vi "Main_spb_framegr.vi"() -> ()   [LabVIEW 2018]
uses:
  <vilib>/Platform/TimedLoop/XDataNode/timing_clust.ctl
  <vilib>/Platform/TimedLoop/XDataNode/nitl_modes.ctl
  <vilib>/Platform/TimedLoop/XDataNode/wakeup.ctl
  <vilib>/rvi/eio/common/nirviEmuTemplateMethod_errors.vi
  <vilib>/rvi/Emulation/niFpgaGetClockAttributes.vi
  <vilib>/rvi/Emulation/niFpgaSctlEmulationGetInTimedLoop.vi
  <vilib>/rvi/Emulation/niFpgaEmulationReportErrorSimple.vi
  <vilib>/rvi/Emulation/niFpgaProcessEmulError.vi
  <vilib>/rvi/Emulation/niFpgaCriticalErrorInLSC.vi
  <vilib>/eio/EIONode/EIONode.xnode
  <vilib>/Platform/TimedLoop/XDataNode/XDataNode.xnode
  <vilib>/Platform/TimedLoop/XDataNode/XDNodeRunTimeDep.lvlib
panel:
  in  "Фильм":bool
  in  "6":i8=6
  in  "12":i8=12
  in  "3":i8=3
  in  "RELAY_18_IN1":bool
  in  "RELAY_18_IN2":bool
  in  "RELAY_28_IN1":bool
  in  "RELAY_28_IN2":bool
  in  "RELAY_30_IN1":bool
  in  "RELAY_30_IN2":bool
  out "I":i32
  in  "Свет до":u32
  in  "Свет от":u32
  in  "Задержка":u32
  in  "Линейки":bool
  in  "Свет":bool
  in  "Строка триггер":u16=1200
  in  "Остановка основного цикла":bool
  in  "Горизонталы":i32=1048
  in  "H1_1":i8=10
  in  "H1_2":i8=36
  in  "H2_1":i8=3
  in  "H2_2":i8=28
  in  "H3_1":i8=20
  in  "H3_2":i8=45
  in  "RG_1":i8=6
  in  "RG_2":i8=16
  in  "48":i8=48
  in  "После H, мкс":u16=15
  in  "CDS1_1":i8=20
  in  "CDS1_2":i8=24
  in  "CDS2_1":i8=36
  in  "CDS2_2":i8=47
  in  "ADC_1":i8=20
  in  "ADC_2":i8=41
  in  "Задержка после переноса строки, мкс":u16=15
  in  "1800":i16=1800
  in  "S3_1":i16=50
  in  "S3_2":i16=950
  in  "S2_1":i16=600
  in  "S2_2":i16=1500
  in  "S1_1":i16=300
  in  "S1_2":i16=1200
  in  "Сколько строк?":i32=2047
  in  "Read(T)/Write(F)":bool
  in  "Enum":T1(ring)
  in  "Write Data":bool[](array[boolean])=[FALSE, FALSE, FALSE, FALSE, FALSE, FALSE, FALSE, FALSE, FALSE]
  in  "8":i8=8
  out "READ":bool[](array[boolean])
  in  "18":i8=18
  in  "7":i8=7
  in  "18_1":i8=18
  in  "Конфигурация":bool
  in  "Кадр":bool
  in  "Command array":bool[](array[boolean])=[FALSE, FALSE, FALSE, FALSE, FALSE, FALSE, FALSE, FALSE, FALSE, FALSE, FALSE, FALSE, FALSE, FALSE, FALSE, FALSE, FALSE]
  # "Чтобы записать кадр в память,\nсначала \"Кадр в память\", затем\nкнопка \"Автомат\""
  # "8"
  # "0"
  # "8"
  # "0"
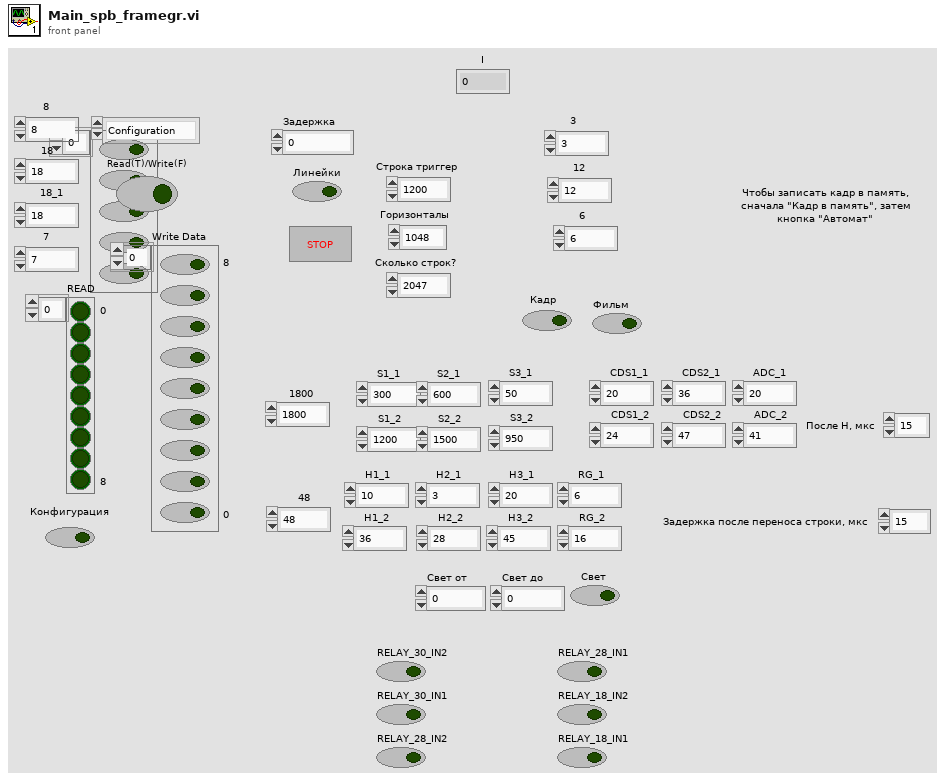
[diagram p1: front panel]
types:
  T1 = enum16{"Configuration", "MUX", "RED PGA", "GREEN PGA", "BLUE PGA", "RED OFF", "GREEN OFF", "BLUE OFF"}
  T2 = typedef "XDNodeRunTimeDep.lvlib/timing_clust.ctl" = cluster{"Expected End [f-1]":u64, "Actual End [f-1]":u64, "Finished Late? [f-1]":bool, "Expected End [i-1]":u64, "Actual End [i-1]":u64, "Finished Late? [i-1]":bool, "Expected Start [i]":u64, "Actual Start [i]":u64, "Expected Start [f]":u64, "Actual Start [f]":u64, "Source Name":string, "Structure Name":string, "Period":i64, "Deadline":i64, "Offset":i64, "Start":i64, "Priority":i32, "Timeout":i32, "Mode":T3, "Wakeup Reason":T4, "Error":errorcluster, "Source Type":string, "Secondary Source Type":string, "Global End Time":u64, "Global Start Time":u64, "Frame Duration":u64, "Iteration Duration":u64, "Assigned CPU":i32, "I/O Scan Engine Mode":u32}
  T3 = typedef "XDNodeRunTimeDep.lvlib/nitl_modes.ctl" = enum32{"No Change", "Process missed periods, maintain original phase", "Discard missed periods, maintain original phase", "Process missed periods, ignore original phase", "Discard missed periods, ignore original phase"}
  T4 = typedef "XDNodeRunTimeDep.lvlib/wakeup.ctl" = enum32{"Normal", "Aborted", "Asynchronous wakeup", "Timing source error", "Timed loop error", "Timeout"}
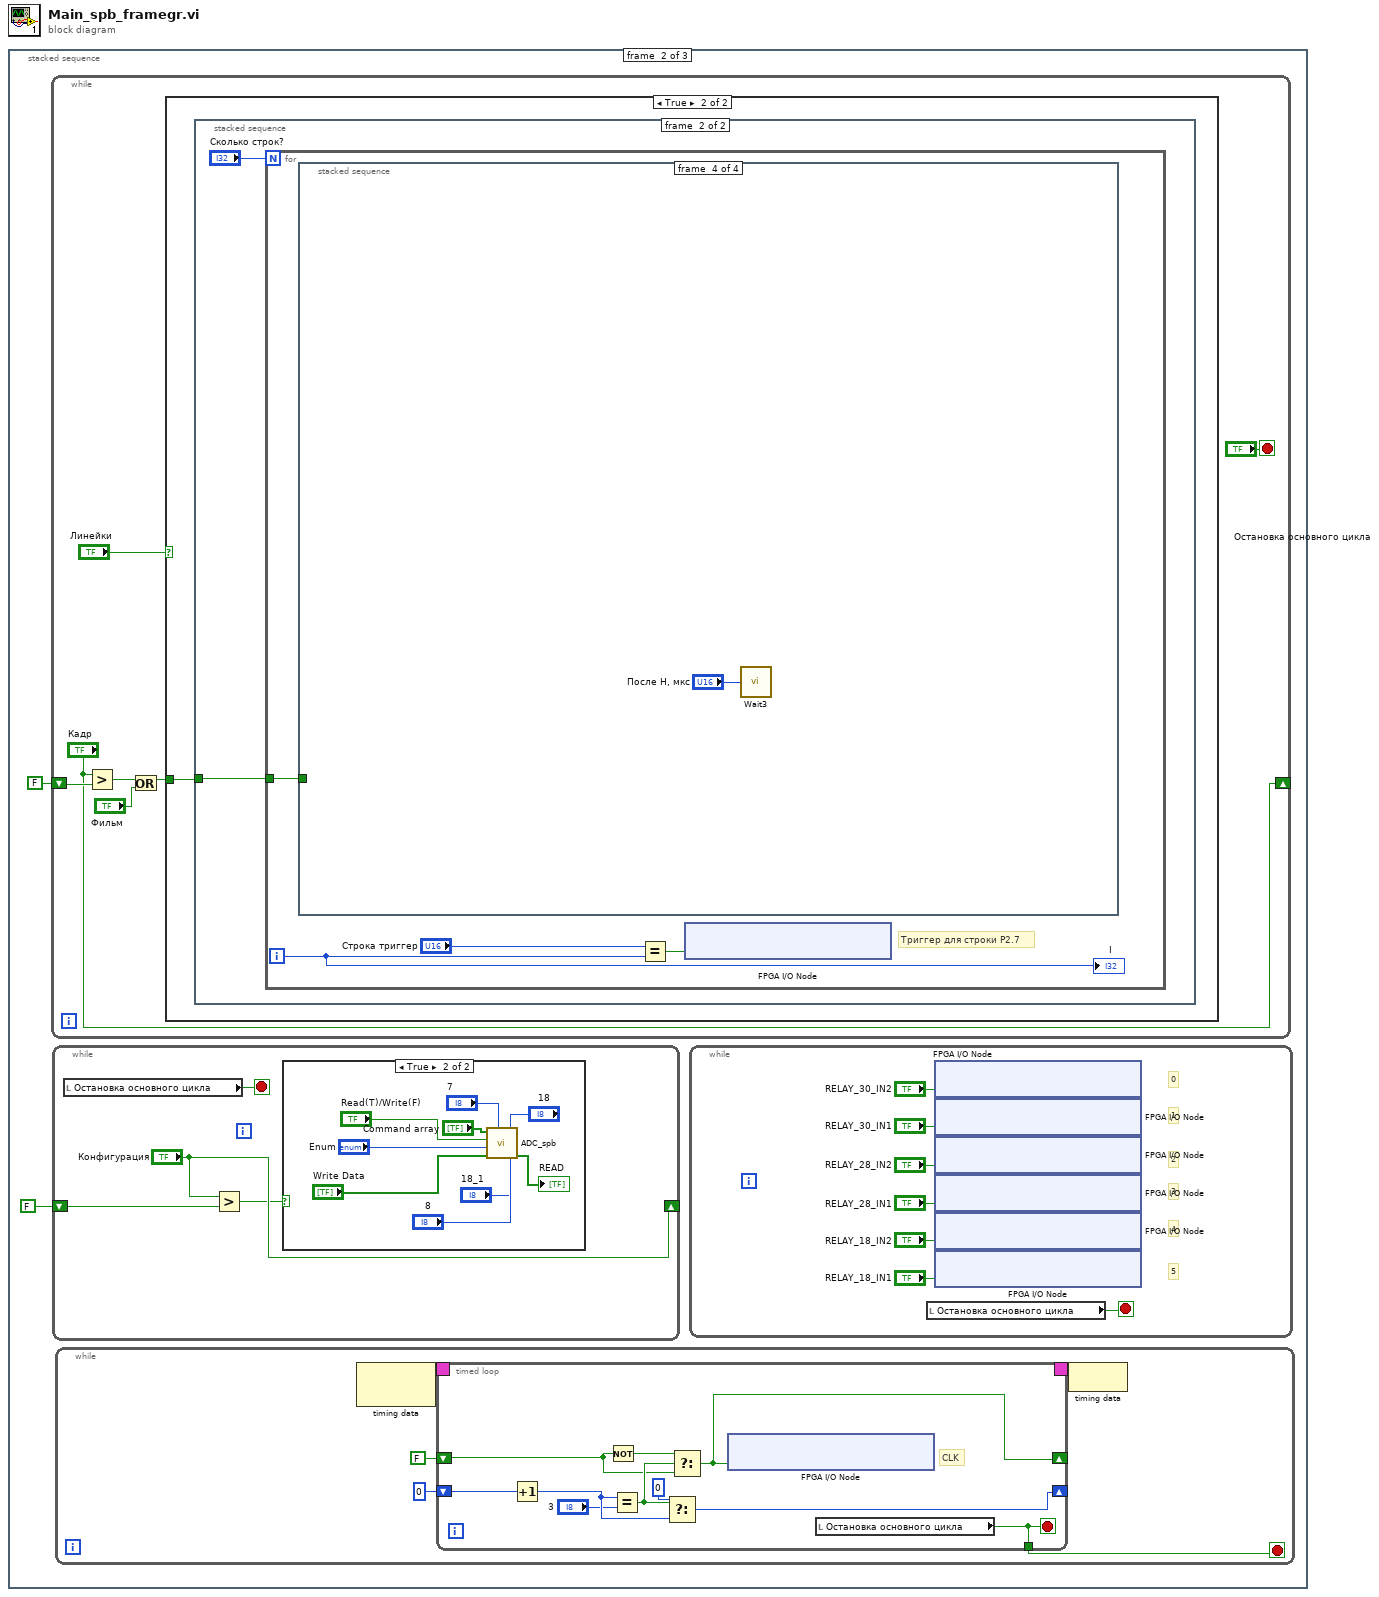
[diagram p0: block diagram]
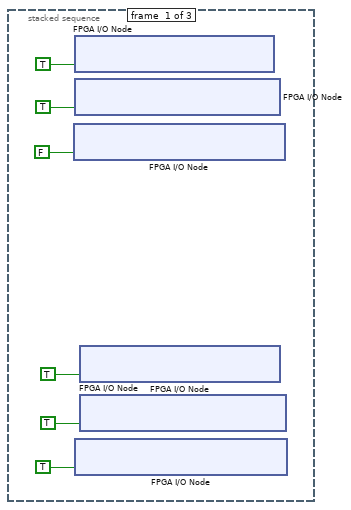
[diagram p2: hidden frame]
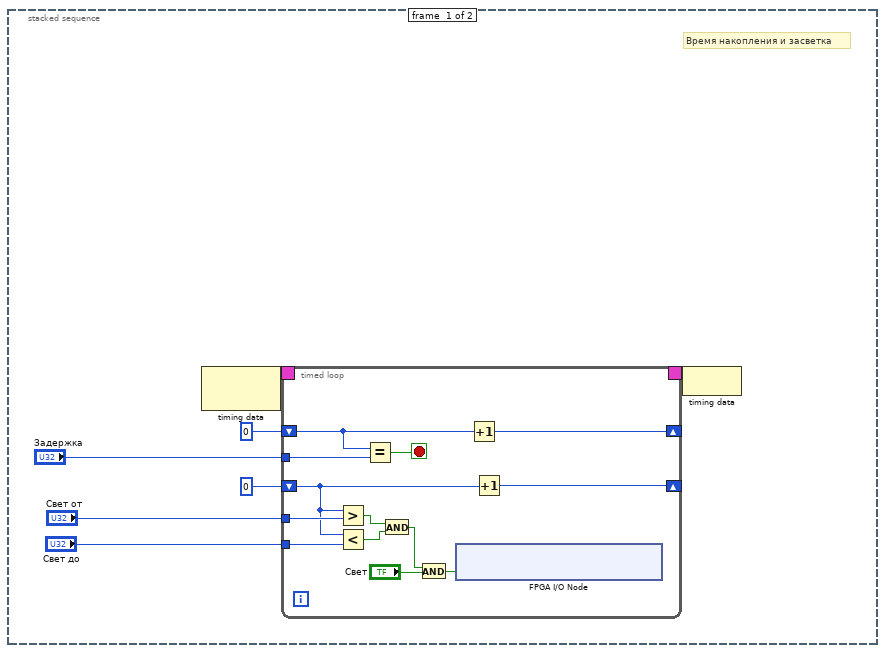
[diagram p4: hidden frame]
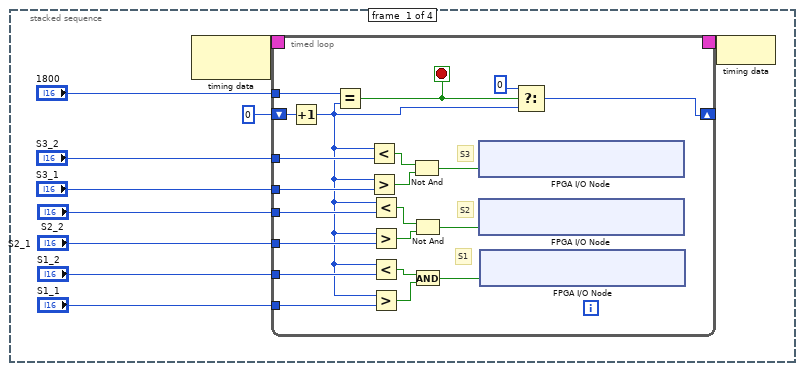
[diagram p5: hidden frame]
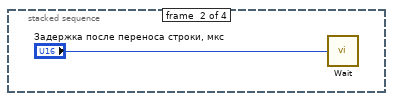
[diagram p6: hidden frame]
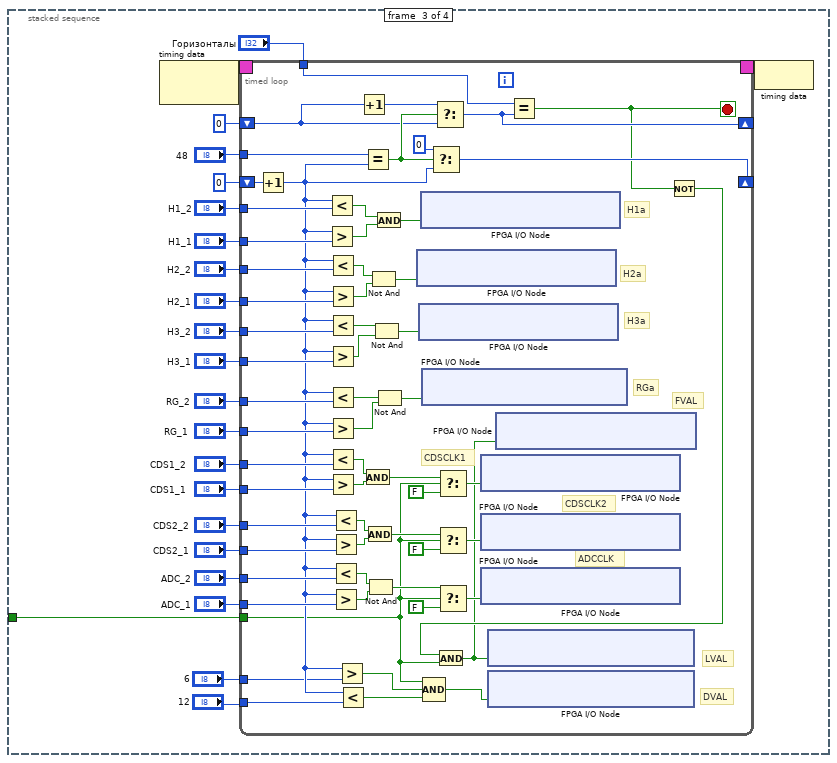
[diagram p7: hidden frame]
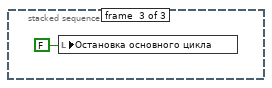
[diagram p9: hidden frame]
diagram:
  n1 = stacked-sequence {
    frame #0 {
      n2 = xnode "FPGA I/O Node"("IO Module\\DDCB_DIO16-23_WE"=FALSE ("IO Module\\DDCB_DIO16-23_WE")) -> ()  [unwired: 1 in, 1 out]
      n3 = xnode "FPGA I/O Node"("IO Module\\DDCB_DIO0-7_WE"=TRUE) -> ()  [unwired: 1 in, 1 out]
      n4 = xnode "FPGA I/O Node"("IO Module\\DDCB_DIO8-15_WE"=TRUE) -> ()  [unwired: 1 in, 1 out]
      n5 = xnode "FPGA I/O Node"("IO Module\\DDCA_DIO16-23_WE"=TRUE) -> ()  [unwired: 1 in, 1 out]
      n6 = xnode "FPGA I/O Node"("IO Module\\DDCA_DIO0-7_WE"=TRUE) -> ()  [unwired: 1 in, 1 out]
      n7 = xnode "FPGA I/O Node"("IO Module\\DDCA_DIO8-15_WE"=TRUE) -> ()  [unwired: 1 in, 1 out]
    }
    frame #1 {
      n8 = while {
        shift-right: ["Кадр"] -> _
        shift-left: FALSE ("Кадр в память") -> [w39]
        stop <- "Остановка основного цикла" stop-if-true
        n9 = Greater?(x="Кадр", y=w39) -> (0:w37:bool)
        n10 = Or(x=w37, y="Фильм") -> (x .or. y?=w36:bool)
        n11 = case shown="True" "Линейки" {
          tunnel: w36 -> [_ w42]
          frame False {
          }
          frame True {
            n12 = stacked-sequence {
              tunnel: w42 -> [_ w68]
              frame #0 {
                # "Время накопления и засветка"
                n13 = node-c288() -> (w49:T2)  [unwired: 1 in]
                n14 = timed-loop {
                  timing: w49 -> [_]
                  timing-out: [_] -> w48
                  shift-right: [w59] -> _
                  shift-left: u32 0 -> [w60]
                  tunnel: "Задержка" -> [w62]
                  shift-right: [w53] -> _
                  shift-left: u32 0 -> [w54]
                  tunnel: "Свет от" -> [w58]
                  tunnel: "Свет до" -> [w57]
                  stop <- w61 stop-if-true
                  n15 = Greater?(x=w54, y=w58) -> (0:w56:bool)
                  n16 = Less?(x=w54, y=w57) -> (x < y?=w55:bool)
                  n17 = Equal?(x=w60, y=w62) -> (x = y?=w61:bool)
                  n18 = And(x=w56, y=w55) -> (x .and. y?=w51:bool)
                  n19 = And(x=w51, y="Свет") -> (x .and. y?=w52:bool)
                  n20 = xnode "FPGA I/O Node"("IO Module\\DDCA_DIO22_Write"=w52) -> ()  [unwired: 1 in, 1 out]
                  n21 = Increment(x=w60) -> (x+1=w59:u32)
                  n22 = Increment(x=w54) -> (x+1=w53:u32)
                }
                n23 = node-c288(w48) -> ()
              }
              frame #1 {
                n24 = for {
                  N: "Сколько строк?" -> [_]
                  tunnel: w68 -> [w70]
                  i -> [w69]
                  # "Триггер для строки Р2.7"
                  n25 = stacked-sequence {
                    tunnel: w70 -> [_ _ w111 _]
                    frame #0 {
                      n26 = node-c288() -> (w82:T2)  [unwired: 1 in]
                      n27 = timed-loop {
                        shift-right: [w101] -> _
                        shift-left: i16 0 -> [w103]
                        timing: w82 -> [_]
                        timing-out: [_] -> w81
                        tunnel: "1800" -> [w100]
                        tunnel: "S3_2" -> [w90]
                        tunnel: "S3_1" -> [w89]
                        tunnel: "S2_2" -> [w88]
                        tunnel: "S2_1" -> [w87]
                        tunnel: "S1_2" -> [w86]
                        tunnel: "S1_1" -> [w85]
                        stop <- w84 stop-if-true
                        # "S1"
                        # "S2"
                        # "S3"
                        n28 = Increment(x=w103) -> (x+1=w83:i16)
                        n29 = Equal?(x=w100, y=w83) -> (x = y?=w84:bool)
                        n30 = Less?(x=w83, y=w90) -> (x < y?=w94:bool)
                        n31 = Greater?(x=w83, y=w89) -> (0:w95:bool)
                        n32 = Less?(x=w83, y=w88) -> (x < y?=w96:bool)
                        n33 = Greater?(x=w83, y=w87) -> (0:w97:bool)
                        n34 = Less?(x=w83, y=w86) -> (x < y?=w98:bool)
                        n35 = Greater?(x=w83, y=w85) -> (0:w99:bool)
                        n36 = Not And(1:w95, 2:w94) -> (0:w93:bool)
                        n37 = Not And(1:w97, 2:w96) -> (0:w92:bool)
                        n38 = And(x=w98, y=w99) -> (x .and. y?=w91:bool)
                        n39 = xnode "FPGA I/O Node"("IO Module\\DDCB_DIO11_Write"=w93) -> ()  [unwired: 1 in, 1 out]
                        n40 = xnode "FPGA I/O Node"("IO Module\\DDCB_DIO12_Write"=w92) -> ()  [unwired: 1 in, 1 out]
                        n41 = xnode "FPGA I/O Node"("IO Module\\DDCB_DIO13_Write"=w91) -> ()  [unwired: 1 in, 1 out]
                        n42 = Select(t=i16 0, s=w84, f=w83) -> (s? t:f=w101:i16)
                      }
                      n43 = node-c288(w81) -> ()
                    }
                    frame #1 {
                      n44 = call "Wait"("Count(uSec)"="Задержка после переноса строки, мкс") -> ()  [unwired: 1 out]
                    }
                    frame #2 {
                      n45 = node-c288() -> (w131:T2)  [unwired: 1 in]
                      n46 = timed-loop {
                        timing: w131 -> [_]
                        timing-out: [_] -> w130
                        tunnel: "H1_2" -> [w187]
                        tunnel: "H1_1" -> [w186]
                        tunnel: "H2_2" -> [w191]
                        tunnel: "H2_1" -> [w190]
                        tunnel: "H3_2" -> [w189]
                        tunnel: "H3_1" -> [w188]
                        shift-right: [w180] -> _
                        shift-left: i8 0 -> [w185]
                        tunnel: "RG_2" -> [w184]
                        tunnel: "RG_1" -> [w183]
                        tunnel: "48" -> [w182]
                        tunnel: "Горизонталы" -> [w164]
                        shift-right: [w163] -> _
                        shift-left: 0 -> [w165]
                        tunnel: "CDS1_2" -> [w156]
                        tunnel: "CDS1_1" -> [w155]
                        tunnel: "CDS2_2" -> [w154]
                        tunnel: "CDS2_1" -> [w153]
                        tunnel: "ADC_2" -> [w152]
                        tunnel: "ADC_1" -> [w151]
                        tunnel: w111 -> [w135]
                        tunnel: "6" -> [w138]
                        tunnel: "12" -> [w137]
                        stop <- w134 stop-if-true
                        # "FVAL"
                        # "LVAL"
                        # "DVAL"
                        # "ADCCLK"
                        # "CDSCLK2"
                        # "CDSCLK1"
                        # "H3a"
                        # "H2a"
                        # "H1a"
                        # "RGa"
                        n47 = Increment(x=w185) -> (x+1=w139:i8)
                        n48 = Less?(x=w139, y=w187) -> (x < y?=w179:bool)
                        n49 = Greater?(x=w139, y=w186) -> (0:w178:bool)
                        n50 = Less?(x=w139, y=w191) -> (x < y?=w177:bool)
                        n51 = Greater?(x=w139, y=w190) -> (0:w176:bool)
                        n52 = Less?(x=w139, y=w189) -> (x < y?=w175:bool)
                        n53 = Greater?(x=w139, y=w188) -> (0:w174:bool)
                        n54 = Less?(x=w139, y=w184) -> (x < y?=w173:bool)
                        n55 = Greater?(x=w139, y=w183) -> (0:w172:bool)
                        n56 = Less?(x=w139, y=w156) -> (x < y?=w157:bool)
                        n57 = Greater?(x=w139, y=w155) -> (0:w158:bool)
                        n58 = Less?(x=w139, y=w154) -> (x < y?=w160:bool)
                        n59 = Greater?(x=w139, y=w153) -> (0:w159:bool)
                        n60 = Less?(x=w139, y=w152) -> (x < y?=w161:bool)
                        n61 = Greater?(x=w139, y=w151) -> (0:w162:bool)
                        n62 = Greater?(x=w139, y=w138) -> (0:w141:bool)
                        n63 = Less?(x=w139, y=w137) -> (x < y?=w140:bool)
                        n64 = Increment(x=w165) -> (x+1=w166:i32)
                        n65 = Equal?(x=w182, y=w139) -> (x = y?=w167:bool)
                        n66 = And(x=w157, y=w158) -> (x .and. y?=w148:bool)
                        n67 = And(x=w160, y=w159) -> (x .and. y?=w147:bool)
                        n68 = Not And(1:w162, 2:w161) -> (0:w146:bool)
                        n69 = Not And(1:w176, 2:w177) -> (0:w169:bool)
                        n70 = Not And(1:w174, 2:w175) -> (0:w168:bool)
                        n71 = And(x=w179, y=w178) -> (x .and. y?=w170:bool)
                        n72 = Not And(1:w172, 2:w173) -> (0:w171:bool)
                        n73 = xnode "FPGA I/O Node"("IO Module\\DDCB_DIO5_Write"=w169) -> ()  [unwired: 1 in, 1 out]
                        n74 = xnode "FPGA I/O Node"("IO Module\\DDCB_DIO6_Write"=w168) -> ()  [unwired: 1 in, 1 out]
                        n75 = xnode "FPGA I/O Node"("IO Module\\DDCB_DIO4_Write"=w170) -> ()  [unwired: 1 in, 1 out]
                        n76 = xnode "FPGA I/O Node"("IO Module\\DDCB_DIO10_Write"=w171) -> ()  [unwired: 1 in, 1 out]
                        n77 = Compound Arithmetic op=AND(w135, w141, w140) -> (w136:bool)
                        n78 = Select(t=i8 0, s=w167, f=w139) -> (s? t:f=w180:i8)
                        n79 = Select(t=w166, s=w167, f=w165) -> (s? t:f=w163:i32)
                        n80 = Select(t=w148, s=w135, f=FALSE) -> (s? t:f=w150:bool)
                        n81 = Select(t=w147, s=w135, f=FALSE) -> (s? t:f=w149:bool)
                        n82 = Select(t=w146, s=w135, f=FALSE) -> (s? t:f=w142:bool)
                        n83 = xnode "FPGA I/O Node"("IO Module\\DDCB_DIO0_Write"=w150) -> ()  [unwired: 1 in, 1 out]
                        n84 = xnode "FPGA I/O Node"("IO Module\\DDCB_DIO3_Write"=w149) -> ()  [unwired: 1 in, 1 out]
                        n85 = xnode "FPGA I/O Node"("IO Module\\DDCB_DIO1_Write"=w142) -> ()  [unwired: 1 in, 1 out]
                        n86 = xnode "FPGA I/O Node"("IO Module\\DDCA_DIO10_Write"=w136) -> ()  [unwired: 1 in, 1 out]
                        n87 = Equal?(x=w164, y=w163) -> (x = y?=w134:bool)
                        n88 = Not(x=w134) -> (.not. x?=w133:bool)
                        n89 = And(x=w133, y=w135) -> (x .and. y?=w132:bool)
                        n90 = xnode "FPGA I/O Node"("IO Module\\DDCA_DIO12_Write"=w132) -> ()  [unwired: 1 in, 1 out]
                        n91 = xnode "FPGA I/O Node"("IO Module\\DDCA_DIO8_Write"=w132) -> ()  [unwired: 1 in, 1 out]
                      }
                      n92 = node-c288(w130) -> ()
                    }
                    frame #3 {
                      n93 = call "Wait3"("Count(uSec)"="После H, мкс") -> ()  [unwired: 1 out]
                    }
                  }
                  n94 = Equal?(x="Строка триггер", y=w69) -> (x = y?=w71:bool)
                  n95 = xnode "FPGA I/O Node"("IO Module\\DDCA_DIO23_Write"=w71) -> ()  [unwired: 1 in, 1 out]
                  "I" <- w69
                }
              }
            }
          }
        }
      }
      n96 = while {
        shift-right: ["Конфигурация"] -> _
        shift-left: FALSE ("Конфигурация") -> [w199]
        stop <- w200 stop-if-true
        n97 = local read "Остановка основного цикла"() -> (w200:bool)
        n98 = Greater?(x="Конфигурация", y=w199) -> (0:w197:bool)
        n99 = case shown="True" w197 {
          frame False {
          }
          frame True {
            n100 = call "ADC_spb.vi"(1:"18_1"="18", 2:"18_1"="18_1", "8"="8", "7"="7", "Write Data"="Write Data", "Enum"="Enum", "Read(T)/Write(F)"="Read(T)/Write(F)", "Command array"="Command array") -> ("READ"=→"READ":bool[])
          }
        }
      }
      n101 = while {
        stop <- w9 stop-if-true
        n102 = node-c288() -> (w13:T2)  [unwired: 1 in]
        n103 = timed-loop {
          timing: w13 -> [_]
          timing-out: [_] -> w12
          shift-right: [w17] -> _
          shift-left: FALSE -> [w18]
          shift-right: [w15] -> _
          shift-left: i8 0 -> [w16]
          tunnel: [w14] -> w9
          stop <- w14 stop-if-true
          # "CLK"
          n104 = Increment(x=w16) -> (x+1=w22:i8)
          n105 = Not(x=w18) -> (.not. x?=w19:bool)
          n106 = Equal?(x=w22, y="3") -> (x = y?=w20:bool)
          n107 = Select(t=i8 0, s=w20, f=w22) -> (s? t:f=w15:i8)
          n108 = Select(t=w19, s=w20, f=w18) -> (s? t:f=w17:bool)
          n109 = xnode "FPGA I/O Node"("IO Module\\DDCA_DIO14_Write"=w17) -> ()  [unwired: 1 in, 1 out]
          n110 = local read "Остановка основного цикла"() -> (w14:bool)
        }
        n111 = node-c288(w12) -> ()
      }
      n112 = while {
        stop <- w34 stop-if-true
        # "5"
        # "4"
        # "3"
        # "2"
        # "1"
        # "0"
        n113 = local read "Остановка основного цикла"() -> (w34:bool)
        n114 = xnode "FPGA I/O Node"("IO Module\\DDCA_DIO16_Write"="RELAY_30_IN2") -> ()  [unwired: 1 in, 1 out]
        n115 = xnode "FPGA I/O Node"("IO Module\\DDCA_DIO17_Write"="RELAY_30_IN1") -> ()  [unwired: 1 in, 1 out]
        n116 = xnode "FPGA I/O Node"("IO Module\\DDCA_DIO18_Write"="RELAY_28_IN2") -> ()  [unwired: 1 in, 1 out]
        n117 = xnode "FPGA I/O Node"("IO Module\\DDCA_DIO19_Write"="RELAY_28_IN1") -> ()  [unwired: 1 in, 1 out]
        n118 = xnode "FPGA I/O Node"("IO Module\\DDCA_DIO20_Write"="RELAY_18_IN2") -> ()  [unwired: 1 in, 1 out]
        n119 = xnode "FPGA I/O Node"("IO Module\\DDCA_DIO21_Write"="RELAY_18_IN1") -> ()  [unwired: 1 in, 1 out]
      }
    }
    frame #2 {
      n120 = local write "Остановка основного цикла"(FALSE) -> ()
    }
  }
